vi "Climb Teleop.vi"(9 "Axes":dbl[](array[numeric]), 11 "Buttons":bool[](array[boolean])) -> ()   [LabVIEW 2019]
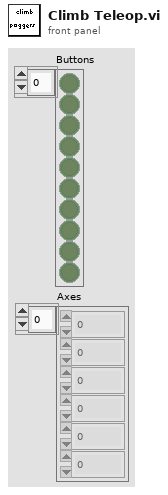
[diagram p1: front panel]
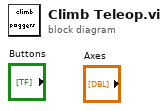
[diagram p0: block diagram]
diagram:
